vi "Rangos.vi"(1 "rangos in":string[](array[string])=["50", "140", "40", "130", "20", "120", "", "", "", "", "", "", "", "", "", "", "", "", "", ""]) -> (0 "rangos out":string[][](array[string]))   [LabVIEW 2019, in "Prueba07.lvclass"]
uses:
  Prueba07.lvclass
panel:
  out "fila":i32
  out "rangos out":string[][](array[string])
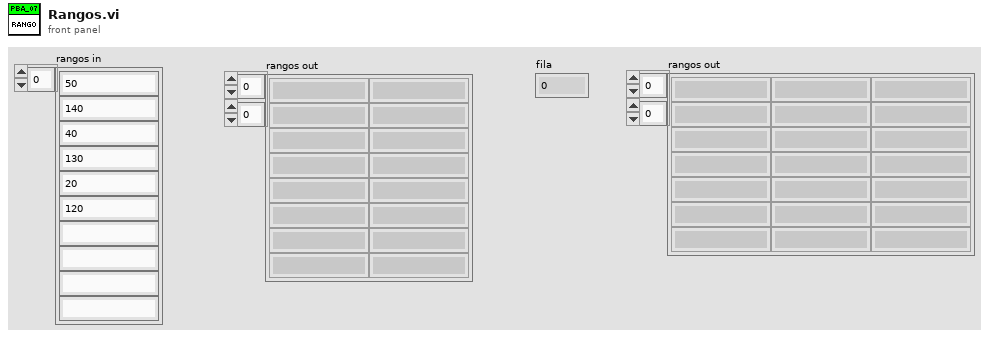
[diagram p1: front panel]
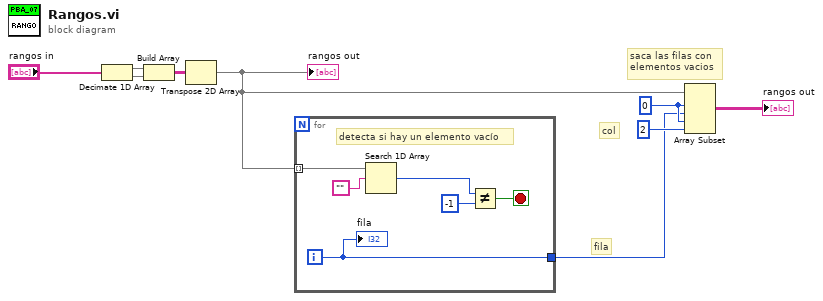
[diagram p0: block diagram]
diagram:
  w3 = 0 ("index")
  # "saca las filas con \nelementos vacios"
  # "fila"
  # "col"
  n1 = Decimate 1D Array("rangos in") -> (w8:string[], w7:string[])
  n2 = Build Array(w8, w7) -> (w6:string[][])
  n3 = Transpose 2D Array(2D array=w6) -> (transposed array=w5:string[][])
  "rangos out" <- w5
  n4 = for {
    tunnel: w5 -> [w15] mode=indexing
    tunnel: [w10] -> w1
    i -> [w10]
    stop <- w11 stop-if-true
    # "detecta si hay un elemento vacío"
    n5 = Search 1D Array(1D array=w15, element="") -> (index of element=w13:i32)  [unwired: 1 in]
    n6 = Not Equal?(x=w13, y=-1) -> (x != y?=w11:bool)
    "fila" <- w10
  }
  n7 = Array Subset(array=w5, index (row)=w3, length (row)=w1, index (col)=w3, length (col)=2 ("length")) -> (→"rangos out":string[][])
